vi "CC Read One Channel from TDMS.vi"(7 "offset (0)":i64, 8 "error in (no error)":errorcluster, 9 "channel":string, 10 "group":string, 11 "tdms file in":refnum<k34>) -> (0 "error out":errorcluster, 1 "timestamps":timestamp[](array[timestamp]), 2 "data":dbl[](array[numeric]), 3 "tdms file out":refnum<k34>, 4 "Units":string)   [LabVIEW 2024]
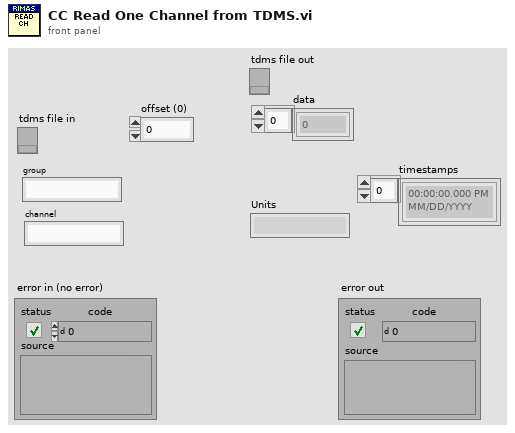
[diagram p1: front panel]
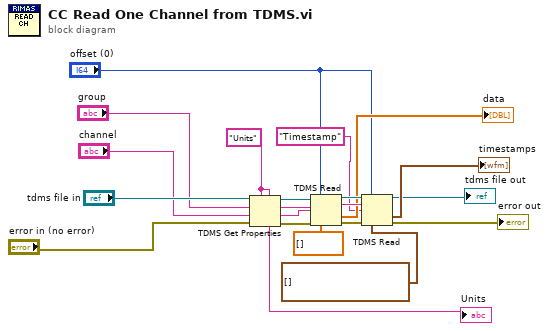
[diagram p0: block diagram]
diagram:
  w9 = "Units" ("property name")
  n1 = TDMS Get Properties(5:w9, 7:w9, 8:"error in (no error)", 9:"channel", 10:"group", 11:"tdms file in") -> (0:w11:errorcluster, 1:w2:string, 2:w3:string, 3:w10:refnum<k34>, 4:→"Units":string)  [unwired: 1 out]
  n2 = TDMS Read(0:w10, 1:"offset (0)", 5:w3, 7:w2, 11:w11, 12:dbl[] []) -> (4:w17:refnum<k34>, 6:w16:string, 10:→"data":dbl[], 15:w15:errorcluster)  [unwired: 2 in, 2 out]
  n3 = TDMS Read(0:w17, 1:"offset (0)", 5:w16, 7:"Timestamp", 11:w15, 12:timestamp[] []) -> (4:→"tdms file out":refnum<k34>, 10:→"timestamps":timestamp[], 15:→"error out":errorcluster)  [unwired: 2 in, 3 out]
